vi "PH_gentec_P-Link.set Measurement Mode.vi"(0 "i ref in":refnum<vi>, 5 "error in":errorcluster) -> (14 "i ref out":refnum<vi>, 19 "error out":errorcluster)   [LabVIEW 2014, in "PH_gentec_P-Link.lvlib"]
doc: "This VI writes wanted Settings to the Device and checks the result."
uses:
  PH_gentec_P-Link.lvlib
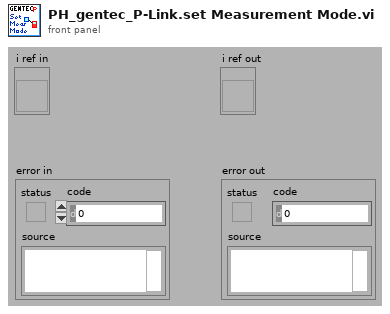
[diagram p1: front panel]
types:
  T1 = typedef "PH_gentec_P-Link.lvlib/PH_gentec_P-Link.i attribute.ctl" = cluster{"GUI References":cluster{"Wanted Head Settings":refnum<vi>, "Current Head Settings":refnum<vi>, "Set Auto Range":refnum<vi>, "Trigger Polarity":refnum<vi>, "Trigger Source":refnum<vi>, "Waveform Averages":refnum<vi>, "Continuous":refnum<vi>, "get one Value":refnum<vi>}, "Wanted Head Settings":T2, "Current Head Settings":T2}
  T2 = typedef "PH_gentec_P-Link.lvlib/PH_gentec_P-Link.Head Settings.ctl" = cluster{"Measurement Mode":T3, "Enable Anticipation":bool, "Set Auto Range":bool, "Block Signal":bool, "Set Head Attenuator":bool, "Enable SSE":bool, "Trigger Polarity":T4, "Trigger Source":T5, "Waveform Averages":T6, "Set Zero":i32, "Current":i32, "Start Data Flow":bool}
  T3 = typedef "gentec-M-Link - Driver.lvlib/gentec-M-Link.Measurement Mode.ctl" = u16
  T4 = typedef "gentec-M-Link - Driver.lvlib/gentec-M-Link.Trigger Polarity.ctl" = u16
  T5 = typedef "gentec-M-Link - Driver.lvlib/gentec-M-Link.Trigger Source.ctl" = u16
  T6 = typedef "gentec-M-Link - Driver.lvlib/gentec-M-Link.Waveform Averages.ctl" = u16
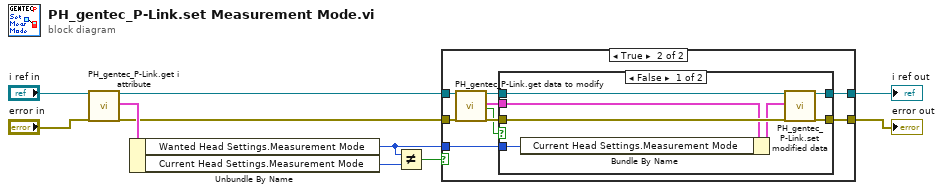
[diagram p0: block diagram]
diagram:
  n1 = call "PH_gentec_P-Link.get i attribute.vi"("i ref in"="i ref in", "error in (no error)"="error in") -> ("i ref out"=w3:refnum<vi>, "i attribute"=w6:T1, "error out"=w5:errorcluster)  [unwired: 15 in]
  n2 = Unbundle By Name(w6) -> ("Wanted Head Settings.Measurement Mode"=w8:T3, "Current Head Settings.Measurement Mode"=w7:T3)
  n3 = Not Equal?(x=w8, y=w7) -> (x != y?=w1:bool)
  n4 = case shown="True" w1 {
    tunnel: [w11 w21] -> w10
    tunnel: [w12 w20] -> w9
    tunnel: w8 -> [_ w19]
    tunnel: w5 -> [w11 w14]
    tunnel: w3 -> [w12 w13]
    frame False {
    }
    frame True {
      n5 = call "PH_gentec_P-Link.get data to modify.vi"("i ref in"=w13, "error in (no error)"=w14) -> ("i ref out"=w17:refnum<vi>, "i attribute"=w16:T1, "timed out"=w15:bool, "error out"=w18:errorcluster)  [unwired: 14 in]
      n6 = case shown="False" w15 {
        tunnel: [w24 w30] -> w20
        tunnel: [w23 w29] -> w21
        tunnel: w18 -> [w27 w29]
        tunnel: w17 -> [w28 w30]
        tunnel: w16 -> [w26 _]
        tunnel: w19 -> [w25 _]
        frame False {
          n7 = Bundle By Name(cluster=w26, "Current Head Settings.Measurement Mode"=w25) -> (w22:T1)
          n8 = call "PH_gentec_P-Link.set modified data.vi"("i ref in"=w28, "i attribute"=w22, "error in (no error)"=w27) -> ("i ref out"=w24:refnum<vi>, "error out"=w23:errorcluster)  [unwired: 15 in]
        }
        frame True {
        }
      }
    }
  }
  "error out" <- w10
  "i ref out" <- w9
